vi "Transport Value.vi"(8 "error in (no error)":errorcluster, 9 "Publish Time":timestamp, 10 "Value":variant, 11 "ISubscriptionPolicy in":refnum<class "ISubscriptionPolicy.lvclass">) -> (0 "error out":errorcluster, 3 "ISubscriptionPolicy out":refnum<class "ISubscriptionPolicy.lvclass">)   [LabVIEW 2019, in "IMediator.lvlib" / "ISubscriptionPolicy.lvclass"]
uses:
  <vilib>/gpm_packages/@cs/mva-core/Source/IMediator/ISubscriptionPolicy/ISubscriptionPolicy.lvclass
  <vilib>/gpm_packages/@cs/mva-core/Source/IMediator/ISubscriptionPolicy/ISubscriptionPolicy.lvclass/ISubscriptionPolicy.ctl
  <vilib>/gpm_packages/@cs/transport/Source/ITransport/ITransport.lvclass
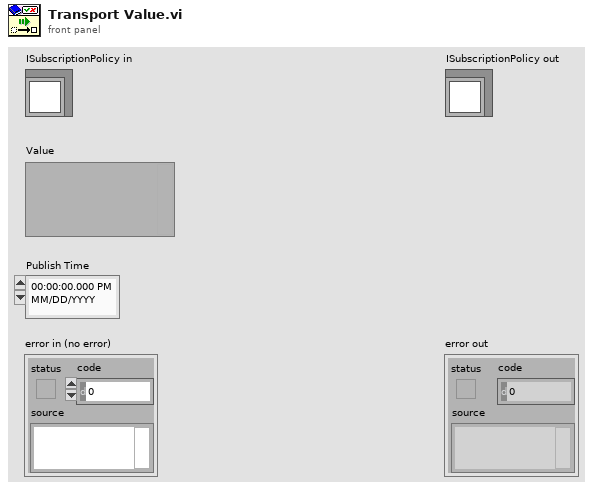
[diagram p1: front panel]
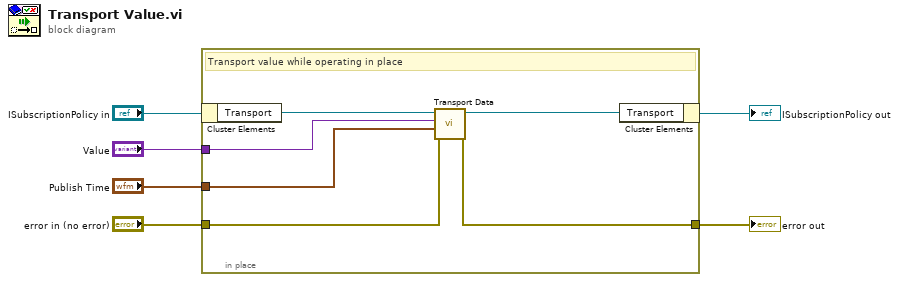
[diagram p0: block diagram]
diagram:
  n1 = in-place {
    in-place-border: "Value" -> [w10]
    in-place-border: "Publish Time" -> [w9]
    in-place-border: "error in (no error)" -> [w8]
    in-place-border: [w7] -> w1
    # "Transport value while operating in place"
    n2 = in-place-cluster #1("ISubscriptionPolicy in") -> ("Transport"=w12:refnum<class "ITransport.lvclass">)
    n3 = call <vilib>:"Transport Data.vi"("error in (no error)"=w8, "Publication Time (Get Time)"=w9, "Value"=w10, "ITransport in"=w12) -> ("error out"=w7:errorcluster, "ITransport out"=w11:refnum<class "ITransport.lvclass">)  [unwired: 6 in]
    n4 = in-place-cluster #1("Transport"=w11) -> (→"ISubscriptionPolicy out":refnum<class "ISubscriptionPolicy.lvclass">)
  }
  "error out" <- w1
